vi "Zip file Handler (from examples).vi"(10 "Source File/Directory":path, 11 "Target Zip File":path) -> ()   [LabVIEW 2010]
panel:
  out "Directory Tree":string(tree)
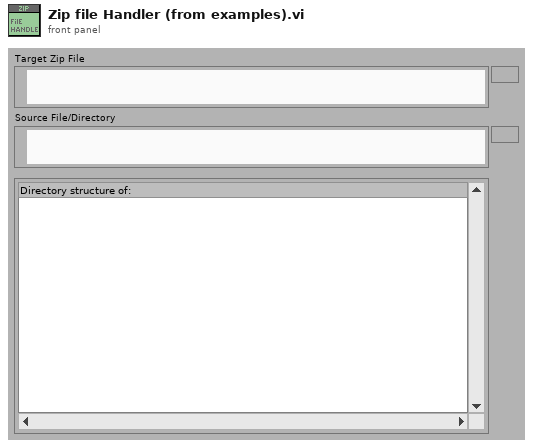
[diagram p1: front panel]
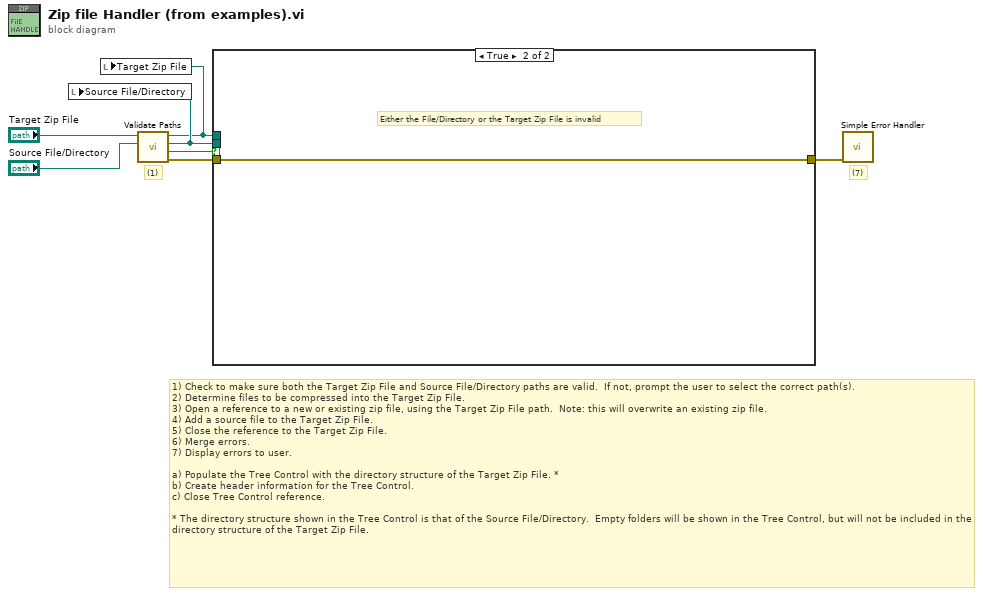
[diagram p0: block diagram]
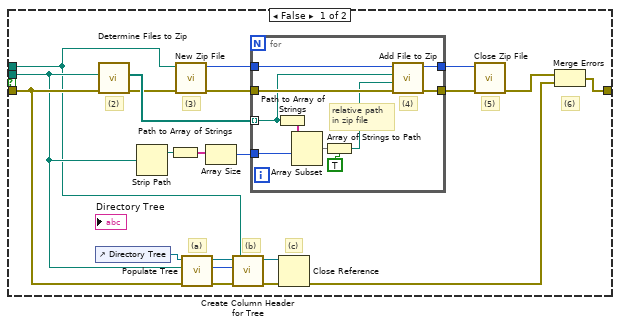
[diagram p2: hidden frame]
diagram:
  # "(7)"
  # "1) Check to make sure both the Target Zip File and Source File/Directory paths are valid.  If not, prompt the user to select the correct path(s).\n2) Determine files to be compressed into the Target Zip File.\n3) Open a reference to a new or existing zip file, using the Target Zip File path.  Note: this will overwrite an existing zip file.\n4) Add a source file to the Target Zip File.\n5) Close the reference to the Target Zip File.\n6) Merge errors.\n7) Display errors to user.\n\na) Populate the Tree Control with the directory structure of the Target Zip File. *\nb) Create header information for the Tree Control.\nc) Close Tree Control reference.\n\n* The directory structure shown in the Tree Control is that of the Source File/Directory.  Empty folders will be shown in the Tree Control, but will not be included in the directory structure of the Target Zip File."
  # "(1)"
  n1 = call "Validate Paths.vi"("File or Directory input"="Source File/Directory", "Target zip file input"="Target Zip File") -> ("error out"=w5:errorcluster, "Invalid Path?"=w4:bool, "File or Directory selected"=w7:path, "Target zip file selected"=w6:path)  [unwired: 6 out]
  n2 = local write "Source File/Directory"(w7) -> ()
  n3 = local write "Target Zip File"(w6) -> ()
  n4 = case shown="True" w4 {
    tunnel: w7 -> [w9 _]
    tunnel: [w19 w39] -> w2
    tunnel: w5 -> [w18 w39]
    tunnel: w6 -> [w8 _]
    frame False {
      # "(6)"
      # "(c)"
      # "(b)"
      # "(a)"
      # "(5)"
      # "(3)"
      # "(2)"
      n5 = control-ref of="Directory Tree"() -> (w15:refnum<vi>)
      n6 = call "Determine Files to Zip.vi"("error in (no error)"=w18, "File or Directory"=w9) -> ("error out"=w17:errorcluster, "Array"=w23:path[])  [unwired: 8 out]
      n7 = Strip Path(path=w9) -> (stripped path=w26:path)  [unwired: 1 out]
      n8 = Path to Array of Strings(0:w26) -> (2:w25:string[])  [unwired: 1 out]
      n9 = call <vilib>:"New Zip File.vi"("error in (no error)"=w17, "target"=w8) -> ("error out"=w27:errorcluster, "zip file out"=w28:i64)  [unwired: 1 in, 3 out]
      n10 = call "Populate Tree.vi"("error in (no error)"=w18, "File or Directory"=w9, "Directory Tree"=w15) -> ("error out"=w16:errorcluster, "Number of files found"=w13:i32, "Directory Tree dup"=w14:refnum<vi>)  [unwired: 6 out]
      n11 = Array Size(array=w25) -> (size(s)=w24:i32)
      n12 = call "Create Column Header for Tree.vi"("Target zip file"=w8, "error in (no error)"=w16, "Number of Files Found"=w13, "Directory Tree"=w14) -> ("error out"=w11:errorcluster, "Directory Tree dup"=w12:refnum<vi>)  [unwired: 2 in, 4 out]
      n13 = for {
        tunnel: w23 -> [w36] mode=indexing
        tunnel: w28 -> [w38]
        tunnel: w27 -> [w37]
        tunnel: w24 -> [w34]
        tunnel: [w30] -> w22
        tunnel: [w29] -> w21
        # "(4)"
        # "relative path\nin zip file"
        n14 = Path to Array of Strings(0:w36) -> (2:w35:string[])  [unwired: 1 out]
        n15 = Array Subset(array=w35, index=w34) -> (w33:string[])  [unwired: 1 in]
        n16 = Array of Strings to Path(0:w33, 1:TRUE ("relative")) -> (2:w32:path)
        n17 = call <vilib>:"Add File to Zip.vi"("error in (no error)"=w37, "destination path in zip"=w32, "source file path"=w36, "zip file in"=w38) -> ("error out"=w30:errorcluster, "zip file out"=w29:i64)  [unwired: 6 out]
      }
      n18 = Close Reference(reference=w12, error in (no error)=w11) -> (error out=w10:errorcluster)
      n19 = call <vilib>:"Close Zip File.vi"("error in (no error)"=w22, "zip file in"=w21) -> ("error out"=w20:errorcluster)  [unwired: 1 in, 4 out]
      n20 = Merge Errors(w20, w10) -> (w19:errorcluster)
    }
    frame True {
      # "Either the File/Directory or the Target Zip File is invalid"
    }
  }
  n21 = call <vilib>:"Simple Error Handler.vi"("error in (no error)"=w2) -> ()  [unwired: 1 in, 8 out]
